vi "Get Drive Info.vi"(8 "error in (no error)":errorcluster caption="错误输入（无错误）", 11 "DriveInfo 输入":refnum<class "DriveInfo.lvclass"> caption="DNL_LabVIEW Object in") -> (0 "error out":errorcluster caption="错误输出", 2 "DriveInfo":T1 {"DriveType" items=["Unknown", "NoRootDirectory", "Removable", "Fixed", "Network", "CDRom", "Ram"]}, 3 "DriveInfo 输出":refnum<class "DriveInfo.lvclass"> caption="DNL_LabVIEW Object out")   [LabVIEW 2012, in "DriveInfo.lvclass"]
uses:
  DriveInfo.lvclass
  Info.ctl
  DriveInfo.lvclass/DriveInfo.ctl
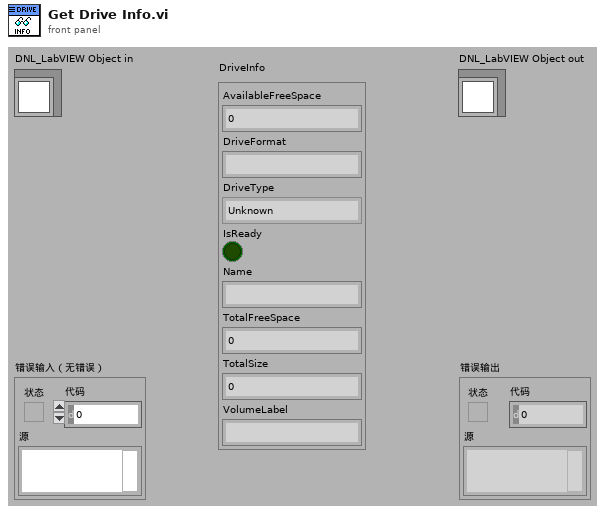
[diagram p1: front panel]
types:
  T1 = typedef "DriveInfo.lvclass/Info.ctl" = cluster{"AvailableFreeSpace":i64, "DriveFormat":string, "DriveType":i32, "IsReady":bool, "Name":string, "TotalFreeSpace":i64, "TotalSize":i64, "VolumeLabel":string}
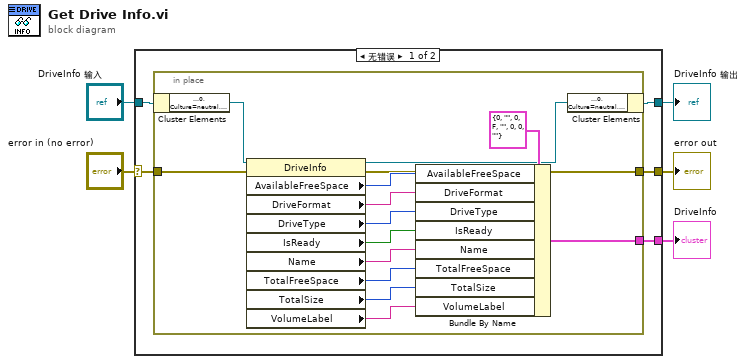
[diagram p0: block diagram]
diagram:
  n1 = case shown="无错误" "error in (no error)" {
    selector: "error in (no error)" -> [w8 w26]
    tunnel: [w7 w26] -> w4
    tunnel: [w6 w25] -> w2
    tunnel: "DriveInfo 输入" -> [w10 w25]
    tunnel: [w9 _] -> w1
    frame No Error {
      n2 = in-place {
        in-place-border: [w21] -> w9
        in-place-border: w8 -> [w19]
        in-place-border: [w18] -> w7
        n3 = in-place-cluster #1(w10) -> ("DriveInfo"=w23:refnum<k24>)
        n4 = property class="DriveInfo"(reference=w23, error in=w19) -> (reference out=w22:refnum<k24>, error out=w18:errorcluster, "AvailableFreeSpace"=w20:i64, "DriveFormat"=w17:string, "DriveType"=w16:i32, "IsReady"=w15:bool, "Name"=w14:string, "TotalFreeSpace"=w13:i64, "TotalSize"=w12:i64, "VolumeLabel"=w11:string)
        n5 = Bundle By Name(cluster=T1 {"AvailableFreeSpace"=0, "DriveFormat"="", "DriveType"=0, "IsReady"=FALSE, "Name"="", "TotalFreeSpace"=0, "TotalSize"=0, "VolumeLabel"=""} ("DriveInfo"), "AvailableFreeSpace"=w20, "DriveFormat"=w17, "DriveType"=w16, "IsReady"=w15, "Name"=w14, "TotalFreeSpace"=w13, "TotalSize"=w12, "VolumeLabel"=w11) -> (w21:T1)
        n6 = in-place-cluster #1("DriveInfo"=w22) -> (w6:refnum<class "DriveInfo.lvclass">)
      }
    }
    frame Error {
    }
  }
  "error out" <- w4
  "DriveInfo 输出" <- w2
  "DriveInfo" <- w1
